vi "FP Show All.vi"(8 "error in (no error)":errorcluster, 11 "DeepU Results in":refnum<class "DeepU Results.lvclass">) -> (0 "error out":errorcluster, 3 "DeepU Results out":refnum<class "DeepU Results.lvclass">)   [LabVIEW 2019, in "Results.lvlib" / "DeepU Results.lvclass"]
uses:
  DeepU Results.lvclass
  DeepU Results.lvclass/DeepU Results.ctl
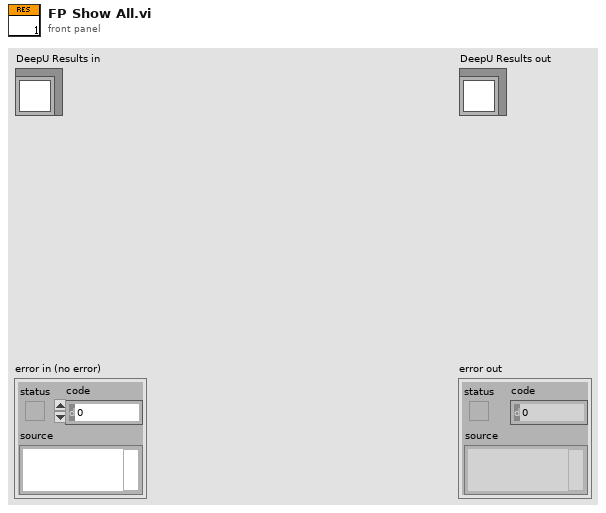
[diagram p1: front panel]
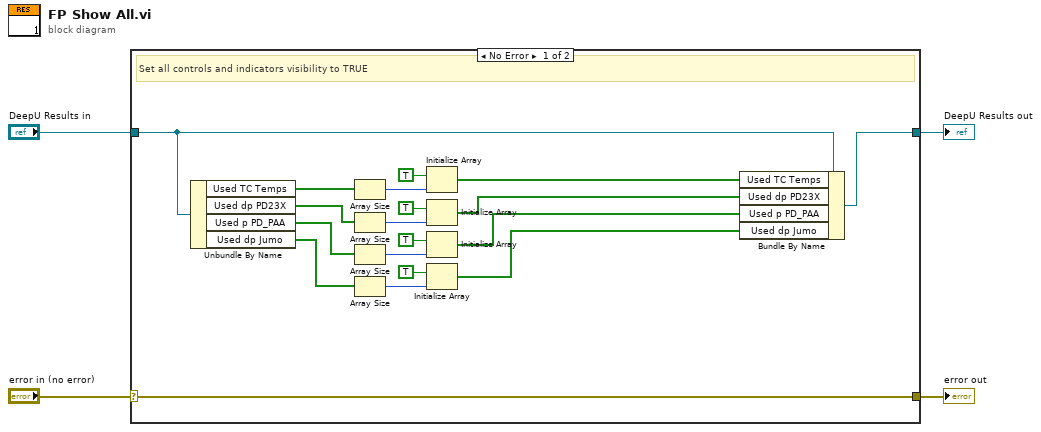
[diagram p0: block diagram]
diagram:
  n1 = case shown="No Error" "error in (no error)" {
    selector: "error in (no error)" -> [w23 w25]
    tunnel: [w23 w25] -> w3
    tunnel: [w22 w24] -> w1
    tunnel: "DeepU Results in" -> [w21 w24]
    frame No Error {
      # "Set all controls and indicators visibility to TRUE"
      n2 = Unbundle By Name(w21) -> ("Used TC Temps"=w20:bool[], "Used dp PD23X"=w15:bool[], "Used p PD_PAA"=w8:bool[], "Used dp Jumo"=w7:bool[])
      n3 = Array Size(array=w20) -> (size(s)=w18:i32)
      n4 = Array Size(array=w15) -> (size(s)=w17:i32)
      n5 = Array Size(array=w8) -> (size(s)=w11:i32)
      n6 = Array Size(array=w7) -> (size(s)=w10:i32)
      n7 = Initialize Array "Initialize Array"(TRUE, w18) -> (w14:bool[])
      n8 = Initialize Array(TRUE, w17) -> (w13:bool[])
      n9 = Initialize Array(TRUE, w11) -> (w6:bool[])
      n10 = Initialize Array(TRUE, w10) -> (w5:bool[])
      n11 = Bundle By Name(cluster=w21, "Used TC Temps"=w14, "Used dp PD23X"=w13, "Used p PD_PAA"=w6, "Used dp Jumo"=w5) -> (w22:refnum<class "DeepU Results.lvclass">)
    }
    frame Error {
    }
  }
  "error out" <- w3
  "DeepU Results out" <- w1
